vi "calc5.vi"() -> ()   [LabVIEW 2010]
uses:
  <instrlib>/niSync/niSync.llb/niSync Initialize (IVI).vi
  <vilib>/Analysis/baseanly.llb/Real Dot Product.vi
  <vilib>/Analysis/NI_AALBase.lvlib
panel:
  out "time":timestamp
  in  "stop":bool
  out "x-y":dbl
  in  "y":string
  in  "x":string
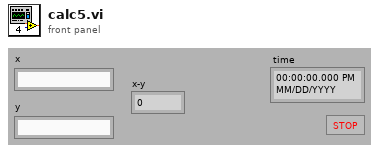
[diagram p1: front panel]
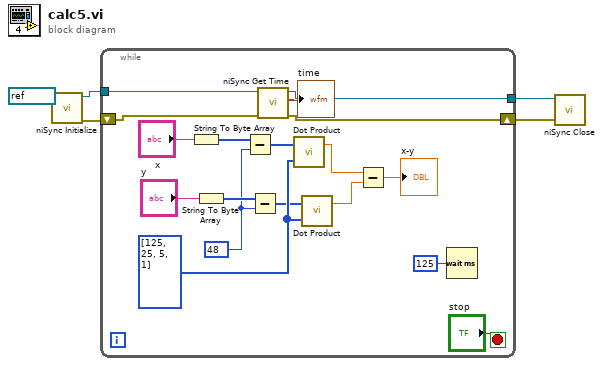
[diagram p0: block diagram]
diagram:
  n1 = call-poly <instrlib>:"niSync Initialize.vi"("resource name"=refnum<k15> "GPS") -> ("error out"=w4:errorcluster, "instrument handle out"=w5:refnum<k15>)  [unwired: 9 in]
  n2 = while {
    tunnel: w5 -> [w10]
    shift-right: [w8] -> w3
    shift-left: w4 -> [w9]
    tunnel: [w7] -> w2
    stop <- "stop" stop-if-true
    w13 = u8 48
    w23 = i32[] [125, 25, 5, 1]
    n3 = String To Byte Array(string="x") -> (unsigned byte array=w18:u8[])
    n4 = String To Byte Array(string="y") -> (unsigned byte array=w19:u8[])
    n5 = Subtract(x=w18, y=w13) -> (x-y=w16:u8[])
    n6 = Subtract(x=w19, y=w13) -> (x-y=w14:u8[])
    n7 = call <instrlib>:"niSync Get Time.vi"("error in (no error)"=w9, "instrument handle"=w10) -> ("error out"=w8:errorcluster, "time"=→"time":timestamp, "instrument handle out"=w7:refnum<k15>)  [unwired: 5 in]
    n8 = call-poly <vilib>:"Dot Product.vi"("Y Vector"=w23, "X Vector"=w16) -> ("X * Y"=w22:dbl)  [unwired: 1 out]
    n9 = call-poly <vilib>:"Dot Product.vi"("Y Vector"=w23, "X Vector"=w14) -> ("X * Y"=w21:dbl)  [unwired: 1 out]
    n10 = Subtract(x=w22, y=w21) -> (x-y=→"x-y":dbl)
    n11 = Wait (ms)(milliseconds to wait=u32 125) -> ()  [unwired: 1 out]
  }
  n12 = call <instrlib>:"niSync Close.vi"("error in (no error)"=w3, "instrument handle"=w2) -> ()  [unwired: 9 in, 1 out]
